vi "Partial_Trace.vi"(8 "error in (no error)":errorcluster, 9 "Qubits to Keep":i32[](array[numeric])=[0, 2, 1], 10 "QuWire in":refnum<class "QuWire.lvclass">, 11 "SimAlg in":refnum<class "PrllPerElmnt.lvclass">) -> (0 "error out":errorcluster, 1 "Reduced Density Matrix":cdb[][](array[numeric]), 2 "QuWire out":refnum<class "QuWire.lvclass">, 3 "SimAlg out":refnum<class "PrllPerElmnt.lvclass">)   [LabVIEW 2020, in "PrllPerElmnt.lvclass"]
uses:
  PrllPerElmnt.lvclass
  QuWire/QuWire.lvclass
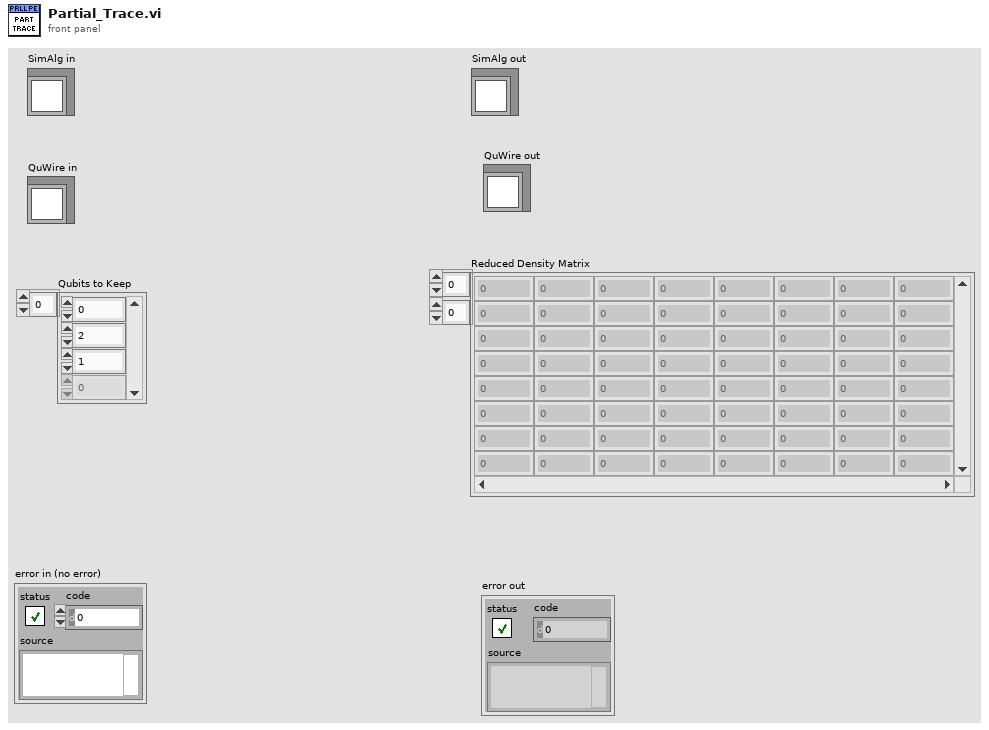
[diagram p1: front panel]
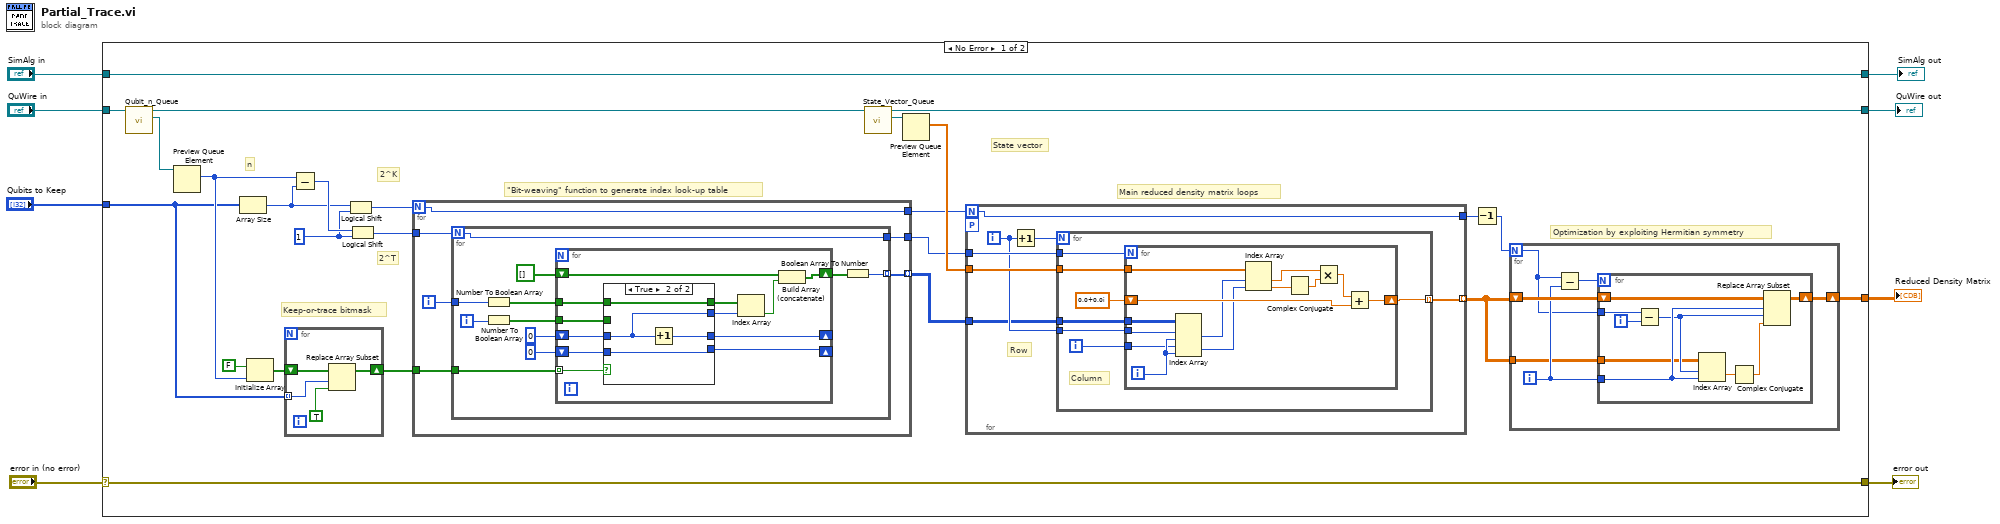
[diagram p0: block diagram]
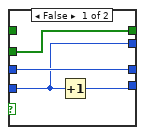
[diagram p2: hidden frame]
diagram:
  n1 = case shown="No Error" "error in (no error)" {
    selector: "error in (no error)" -> [w32 w119]
    tunnel: [w32 w119] -> w7
    tunnel: [w33 w118] -> w5
    tunnel: "SimAlg in" -> [w33 w118]
    tunnel: "QuWire in" -> [w28 w117]
    tunnel: [w27 w117] -> w3
    tunnel: "Qubits to Keep" -> [w20 _]
    tunnel: [w18 _] -> w1
    frame No Error {
      w22 = 1 ("x")
      # "2^T"
      # "2^K"
      # "Main reduced density matrix loops"
      # "\"Bit-weaving\" function to generate index look-up table"
      # "Optimization by exploiting Hermitian symmetry"
      # "Keep-or-trace bitmask"
      # "State vector"
      # "n"
      n2 = call "Qubit_n_Queue.vi"("QuWire in"=w28) -> ("Qubit n"=w30:refnum<queue>, "QuWire out"=w29:refnum<class "QuWire.lvclass">)  [unwired: 8 in, 1 out]
      n3 = Preview Queue Element(queue=w30) -> (element=w21:i32)  [unwired: 2 in, 3 out]
      n4 = Array Size(array=w20) -> (size(s)=w23:i32)
      n5 = Initialize Array(FALSE, w21) -> (w26:bool[])
      n6 = for {
        tunnel: w20 -> [w35] mode=indexing
        shift-right: [w34] -> w14
        shift-left: w26 -> [w37]
        n7 = Replace Array Subset(array=w37, new element=TRUE ("new element/subarray"), index=w35) -> (w34:bool[])
      }
      n8 = Subtract(x=w21, y=w23) -> (x-y=w24:i32)
      n9 = Logical Shift(y=w23, x=w22) -> (x << y=w12:i32)
      n10 = Logical Shift(y=w24, x=w22) -> (x << y=w13:i32)
      n11 = for {
        N: w12 -> [w39]
        tunnel: w14 -> [w43]
        tunnel: w13 -> [w41]
        tunnel: [w40] -> w11 mode=indexing
        tunnel: [w39] -> w10
        tunnel: [w38] -> w9
        i -> [w42]
        n12 = for {
          N: w41 -> [w44]
          tunnel: w43 -> [w48]
          tunnel: w42 -> [w46]
          tunnel: [w45] -> w40 mode=indexing
          tunnel: [w44] -> w38
          i -> [w47]
          n13 = Number To Boolean Array(number=w46) -> (Boolean array=w49:bool[])
          n14 = Number To Boolean Array(number=w47) -> (Boolean array=w52:bool[])
          n15 = for {
            tunnel: w48 -> [w66] mode=indexing
            tunnel: w49 -> [w58]
            tunnel: w52 -> [w65]
            shift-right: [w62] -> w53
            shift-left: bool[] [] -> [w61]
            shift-right: [w63] -> _
            shift-left: 0 -> [w64]
            shift-right: [w56] -> _
            shift-left: 0 -> [w57]
            n16 = case shown="True" w66 {
              tunnel: w65 -> [w67 _]
              tunnel: w64 -> [w70 w73]
              tunnel: [w70 w74] -> w63
              tunnel: [w68 w73] -> w60
              tunnel: [w67 w72] -> w59
              tunnel: w58 -> [_ w72]
              tunnel: w57 -> [w68 w71]
              tunnel: [w69 w71] -> w56
              frame False {
                n17 = Increment(x=w68) -> (x+1=w69:i32)
              }
              frame True {
                n18 = Increment(x=w73) -> (x+1=w74:i32)
              }
            }
            n19 = Index Array(array=w59, index=w60) -> (element=w55:bool)
            n20 = Build Array (concatenate)(w61, w55) -> (w62:bool[])
          }
          n21 = Boolean Array To Number(Boolean array=w53) -> (number=w45:u32)
        }
      }
      n22 = call "State_Vector_Queue.vi"("QuWire in"=w29) -> ("State Vector Queue"=w31:refnum<queue>, "QuWire out"=w27:refnum<class "QuWire.lvclass">)  [unwired: 8 in, 1 out]
      n23 = Preview Queue Element(queue=w31) -> (element=w19:cdb[])  [unwired: 2 in, 3 out]
      n24 = for {
        N: w10 -> [w76]
        tunnel: w19 -> [w81]
        tunnel: w9 -> [w80]
        tunnel: [w78] -> w17 mode=indexing
        tunnel: [w76] -> w16
        tunnel: w11 -> [w75]
        workers-P: _ -> [_]
        i -> [w79]
        # "Row"
        n25 = Increment(x=w79) -> (x+1=w77:i32)
        n26 = for {
          N: w77 -> [_]
          tunnel: w81 -> [w88]
          tunnel: w79 -> [w85]
          tunnel: w80 -> [w86]
          tunnel: [w83] -> w78 mode=indexing
          tunnel: w75 -> [w82]
          i -> [w87]
          # "Column"
          n27 = for {
            N: w86 -> [_]
            tunnel: w88 -> [w101]
            tunnel: w87 -> [w91]
            tunnel: w85 -> [w93]
            shift-right: [w95] -> w83
            shift-left: cdb 0.0+0.0i ("element") -> [w97]
            tunnel: w82 -> [w94]
            i -> [w92]
            n28 = Index Array(array=w94, index (row) #1=w93, index (col) #1=w92, index (row) #2=w91, index (col) #2=w92) -> (element #1=w90:u32, element #2=w89:u32)
            n29 = Index Array(array=w101, index #1=w90, index #2=w89) -> (element #1=w96:cdb, element #2=w100:cdb)
            n30 = Complex Conjugate(1:w100) -> (0:w99:cdb)
            n31 = Multiply(x=w96, y=w99) -> (x*y=w98:cdb)
            n32 = Add(x=w98, y=w97) -> (x+y=w95:cdb)
          }
        }
      }
      n33 = Decrement(x=w16) -> (x-1=w15:i32)
      n34 = for {
        N: w15 -> [w102]
        shift-right: [w105] -> w18
        shift-left: w17 -> [w107]
        tunnel: w17 -> [w103]
        i -> [w104]
        n35 = Subtract(x=w102, y=w104) -> (x-y=w106:i32)
        n36 = for {
          N: w106 -> [_]
          tunnel: w104 -> [w112]
          shift-right: [w116] -> w105
          shift-left: w107 -> [w110]
          tunnel: w103 -> [w109]
          tunnel: w102 -> [w108]
          i -> [w113]
          n37 = Subtract(x=w108, y=w113) -> (x-y=w111:i32)
          n38 = Index Array(array=w109, index (row)=w111, index (col)=w112) -> (element=w115:cdb)
          n39 = Complex Conjugate(1:w115) -> (0:w114:cdb)
          n40 = Replace Array Subset(array=w110, new element=w114, index (row)=w112, index (col)=w111) -> (w116:cdb[][])
        }
      }
    }
    frame Error {
    }
  }
  "error out" <- w7
  "SimAlg out" <- w5
  "QuWire out" <- w3
  "Reduced Density Matrix" <- w1
